vi "playVlc.vi"(8 "error in (no error)":errorcluster, 10 "playVlc":string, 11 "VlcPlayer in":refnum<class "VlcPlayer.lvclass">) -> (0 "error out":errorcluster, 3 "VlcPlayer out":refnum<class "VlcPlayer.lvclass">)   [LabVIEW 2017, in "VlcPlayer.lvclass"]
uses:
  VlcPlayer.lvclass
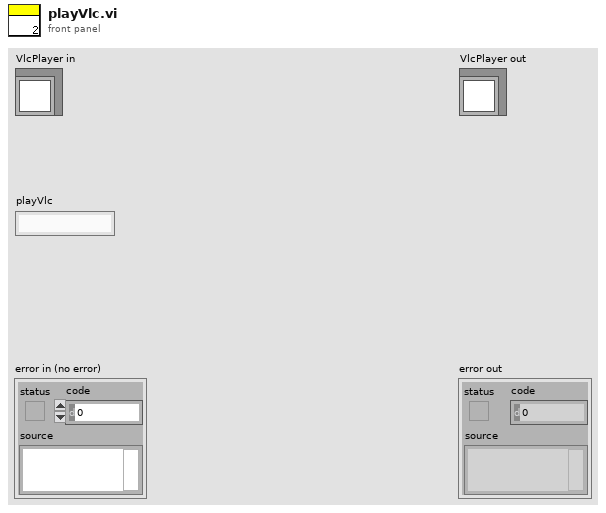
[diagram p1: front panel]
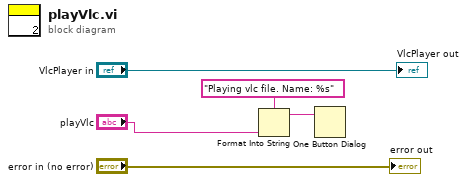
[diagram p0: block diagram]
diagram:
  n1 = Format Into String(format string="Playing vlc file. Name: %s", "playVlc") -> (resulting string=w3:string)  [unwired: 2 in, 1 out]
  n2 = One Button Dialog(message=w3) -> ()  [unwired: 1 in, 1 out]
  "error out" <- "error in (no error)"
  "VlcPlayer out" <- "VlcPlayer in"
